vi "EasyVIAborterAuto.vi"() -> ()   [LabVIEW 2014]
panel:
  in  "Filter Running?":bool=TRUE
  # "Easy VI Aborter"
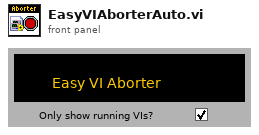
[diagram p1: front panel]
types:
  T1 = enum32{"Bad", "Idle", "Run top level", "Running"}
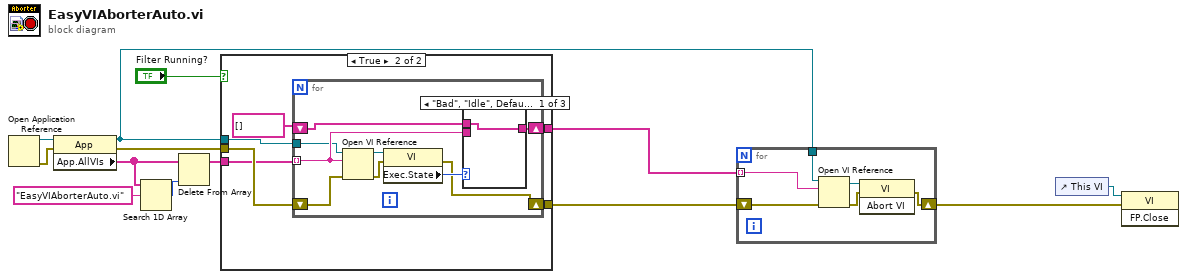
[diagram p0: block diagram]
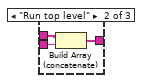
[diagram p3: hidden frame]
diagram:
  n1 = Open Application Reference() -> (0:w10:errorcluster, 3:w11:refnum<vi>)  [unwired: 4 in]
  n2 = property class="App"(reference=w11, error in=w10) -> (reference out=w2:refnum<vi>, error out=w8:errorcluster, "App.AllVIs"=w6:string[])
  n3 = Search 1D Array(1D array=w6, element="EasyVIAborterAuto.vi") -> (index of element=w5:i32)  [unwired: 1 out]
  n4 = Delete From Array(array=w6, index=w5) -> (array with subset deleted=w4:string[])  [unwired: 1 in, 1 out]
  n5 = case shown="True" "Filter Running?" {
    tunnel: [w15 w21] -> w9
    tunnel: [w14 w20] -> w1
    tunnel: w8 -> [w14 w19]
    tunnel: w4 -> [w15 w17]
    tunnel: w2 -> [_ w16]
    frame False {
    }
    frame True {
      n6 = for {
        tunnel: w17 -> [w28] mode=indexing
        shift-right: [w27] -> w21
        shift-left: string[] [] -> [w26]
        shift-right: [w24] -> w20
        shift-left: w19 -> [w23]
        tunnel: w16 -> [w22]
        n7 = Open VI Reference(application reference (local)=w22, vi path=w28, error in (no error)=w23) -> (vi reference=w30:refnum<vi>, error out=w25:errorcluster)  [unwired: 3 out]
        n8 = property class="VI"(reference=w30, error in=w25) -> (error out=w24:errorcluster, "Exec.State"=w29:T1)  [unwired: 1 out]
        n9 = case shown="\"Bad\", \"Idle\", Default" w29 {
          tunnel: w28 -> [_ w33 _]
          tunnel: [w31 w32 w35] -> w27
          tunnel: w26 -> [w31 w34 w35]
          frame "Bad", "Idle", Default {
          }
          frame "Run top level" {
            n10 = Build Array (concatenate)(w34, w33) -> (w32:string[])
          }
          frame "Running" {
          }
        }
      }
    }
  }
  n11 = for {
    tunnel: w9 -> [w36] mode=indexing
    shift-right: [w38] -> w12
    shift-left: w1 -> [w40]
    tunnel: w2 -> [w37]
    n12 = Open VI Reference(application reference (local)=w37, vi path=w36, error in (no error)=w40) -> (vi reference=w41:refnum<vi>, error out=w39:errorcluster)  [unwired: 3 out]
    n13 = invoke class="VI" method="Abort VI"(reference=w41, error in=w39) -> (error out=w38:errorcluster)  [unwired: 1 in, 2 out]
  }
  n14 = control-ref of="This VI"() -> (w13:refnum<vi>)
  n15 = invoke class="VI" method="FP.Close"(reference=w13, error in=w12) -> ()  [unwired: 1 in, 3 out]
